vi "Icai 105 - Simultry11_Current Working Version.vi"() -> ()   [LabVIEW 2010]
uses:
  <vilib>/DAQmx/write.llb/DAQmx Write (Analog 1D Wfm NChan NSamp).vi
  <vilib>/DAQmx/write.llb/DAQmx Write (Digital 1D Bool 1Chan 1Samp).vi
  <vilib>/DAQmx/write.llb/DAQmx Write (Analog Wfm 1Chan NSamp).vi
  <vilib>/Waveform/WDTOps.llb/WDT Append Waveforms DBL.vi
  <vilib>/measure/matone.llb/Extract Single Tone Information 1 Chan.vi
  <vilib>/DAQmx/create/channels.llb/DAQmx Create Channel (DO-Digital Output).vi
  <vilib>/DAQmx/create/channels.llb/DAQmx Create Channel (AO-Voltage-Basic).vi
  <vilib>/DAQmx/configure/timing.llb/DAQmx Timing (Sample Clock).vi
  <vilib>/daqmx/miscellaneous.llb/DAQmx Fill In Error Info.vi
  <vilib>/measure/NI_MABase.lvlib
  <vilib>/measure/NI_MAPro.lvlib
  Program Files/National Instruments/LabVIEW 2010/resource/objmgr/daqmx.rc
panel:
  out "error out 2":errorcluster
  out "number of samples written per channel":u32
  out "detected frequency 2":dbl format="%.6p"
  out "SampClk.Timebase.Rate":dbl format="%^#_10g"
  in  "Freq Scale Factor":dbl=1.0 format="%#_12g"
  out "signal out":waveform(dbl)(graph)
  in  "lines":tag="Dev1/port0/line3"
  in  "Rising Logic Output Chan":tag="Dev1/ao2"
  in  "Mod Duration ms":i32=300
  in  "Samples (1Ms/s)":i32=500000
  out "min value":dbl
  in  "Falling Logic Output Chan":tag="Dev1/ao1"
  in  "FM Waveform Channel":tag="Dev1/ao3"
  out "error out":errorcluster caption="error out (DAQ)"
  out "Mod":dbl=118572.0
  out "Numeric 2":dbl=3900000.0 format="%#_7g"
  out "Numeric":dbl=3900000.0 format="%#_7g"
  in  "Pre-Trig Samples":ext=100.0 format="%.2f"
  out "?":dbl=579698.7113293351 format="%#_6f"
  out "#s":dbl=39524.02451426849
  in  "Time int":i32=30000
  in  "Sensitivity":u16(ring)=19 items=["2 nV/fA", "5 nV/fA", "10 nV/fA", "20 nV/fA", "50 nV/fA", "100 nV/fA", "200 nV/fA", "500 nV/fA", "1 uV/pA", "2 uV/pA", "5 uV/pA", "10 uV/pA", "20 uV/pA", "50 uV/pA", "100 uV/pA", "200 uV/pA", "500 uV/pA", "1 mV/nA", "2 mV/nA", "5 mV/nA", "10 mV/nA", "20 mV/nA", "50 mV/nA", "100 mV/nA", "200 mV/nA", "500 mV/nA", "1 V/uA"]
  in  "Detection Bandwidth":u16(ring)=6 items=["10 us/ 25 kHz", "30 us /8.33 kHz", "100 us/ 2.50 kHz", "300 us/ 833 Hz", "1 ms /250 Hz", "3 ms /83.3 Hz", "10 ms/ 25 Hz", "30 ms/ 8.33 Hz", "100 ms/ 2.50 Hz", "300 ms/ 0.833 Hz ", "1 s/ 0.250 Hz", "3 s/ 0.0833 Hz", "10 s/0.025 Hz"]
  in  "SR 830 GPIB Address":i32=8
  in  "Freq 2":dbl=2447.6 format="%_7g"
  out "Iterat #":dbl=10.0
  in  "Iteration":dbl=500.0
  in  "stop 2":bool
  in  "pulse":bool=TRUE
  in  "Start":ext=0.05
  out "?":waveform(dbl)[](graph)
  in  "amplitude 2":dbl=0.25 format="%0.2p"
  in  "?":T1(ring)
  in  "phase 2":dbl format="%.2p"
  in  "Offset 2":dbl=-0.0 format="%#_6p"
  in  "frequency 4":dbl=100.0 format="%0.2p"
  in  "?":T1(ring)=enum."Triangle Wave"
  in  "offset 4":dbl=-1.0 format="%0.2p"
  in  "phase 4":dbl=90.0 format="%.2p"
  in  "amplitude 4":dbl=1.0 format="%0.2p"
  in  "frequency 1":dbl=100.0 format="%0.2p"
  in  "amplitude 1":dbl=1.0 format="%0.2p"
  in  "sampling info 1":cluster{"Fs":dbl, "#s":dbl}={"Fs"=1000000.0, "#s"=2500.0} {"Fs" format="%.2p"}
  in  "?":T1(ring)=enum."Triangle Wave"
  in  "phase 1":dbl=-90.0 format="%.2p"
  in  "Offset 1":dbl format="%#_6p"
  in  "iterat":dbl
  out "CW":dbl=123571.0
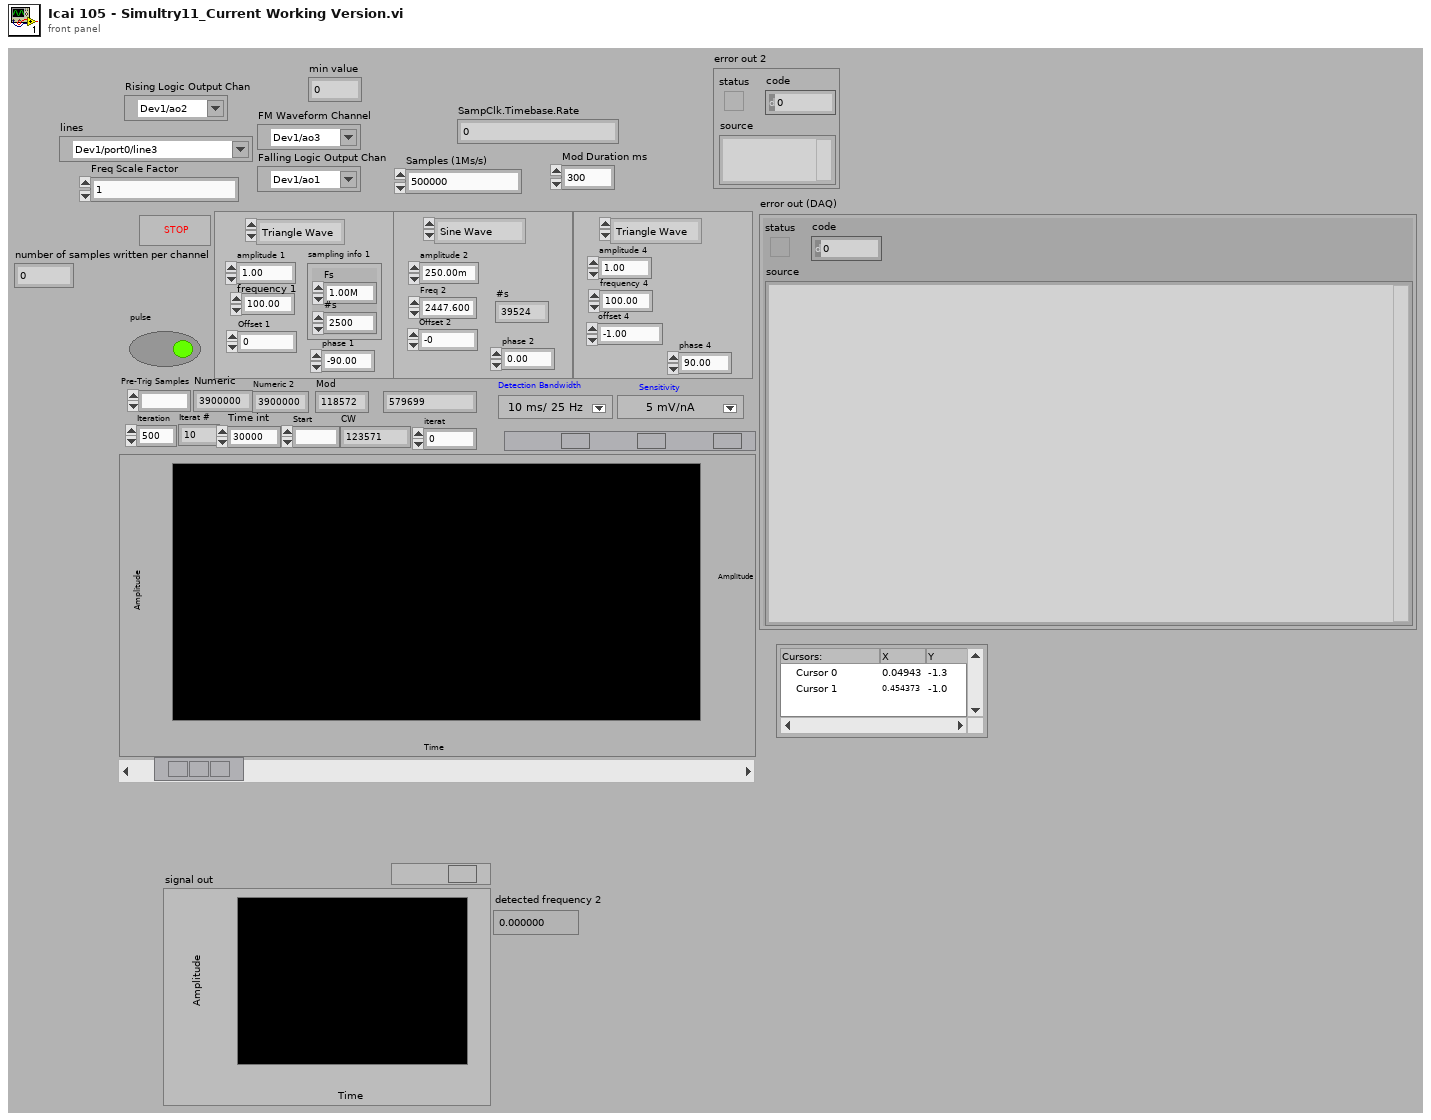
[diagram p1: front panel]
types:
  T1 = enum16{"Sine Wave", "Triangle Wave", "Square Wave", "Sawtooth Wave"}
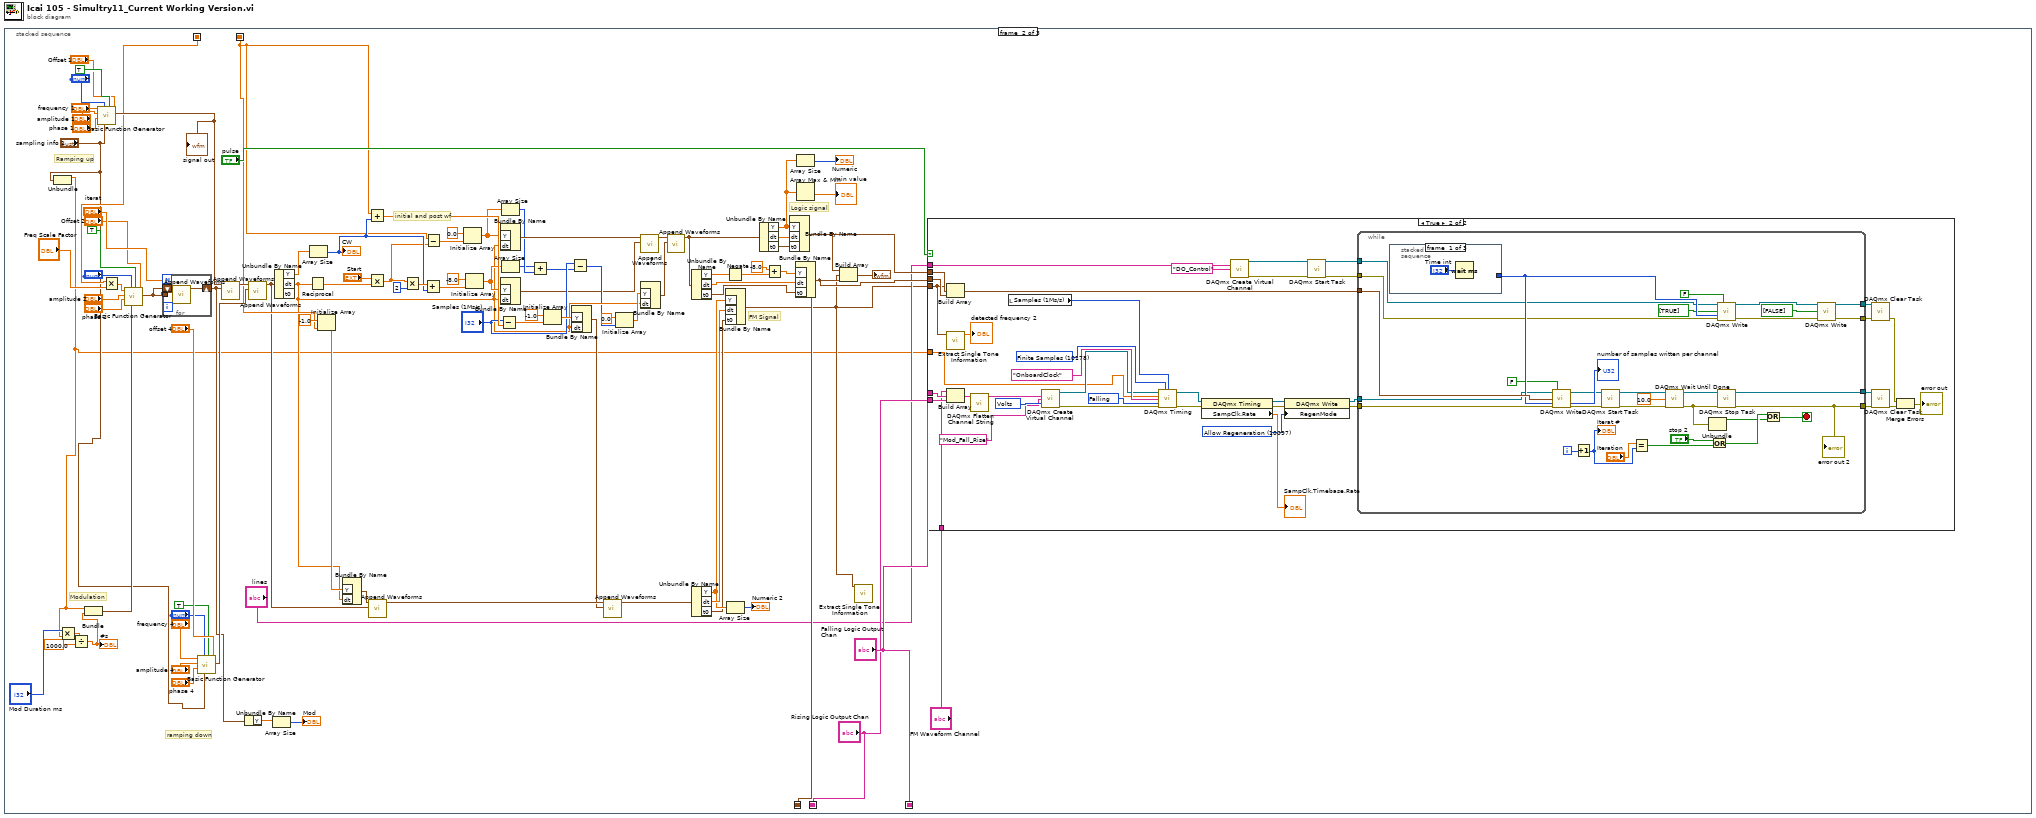
[diagram p0: block diagram]
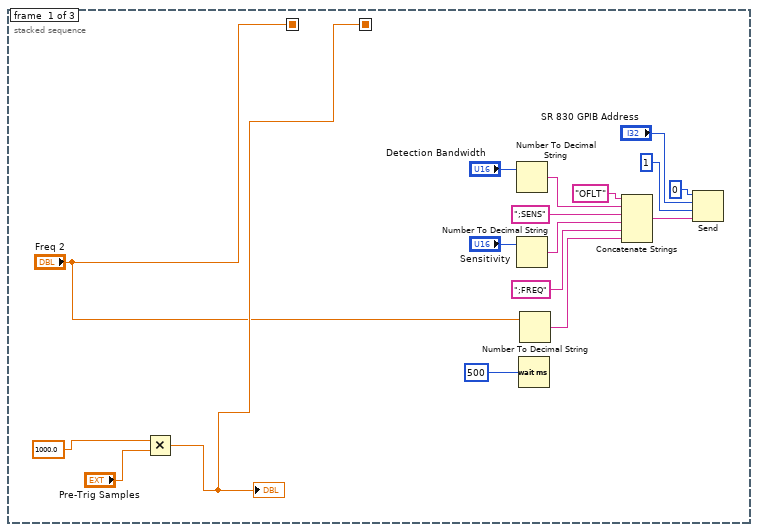
[diagram p2: hidden frame]
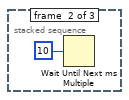
[diagram p4: hidden frame]
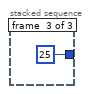
[diagram p5: hidden frame]
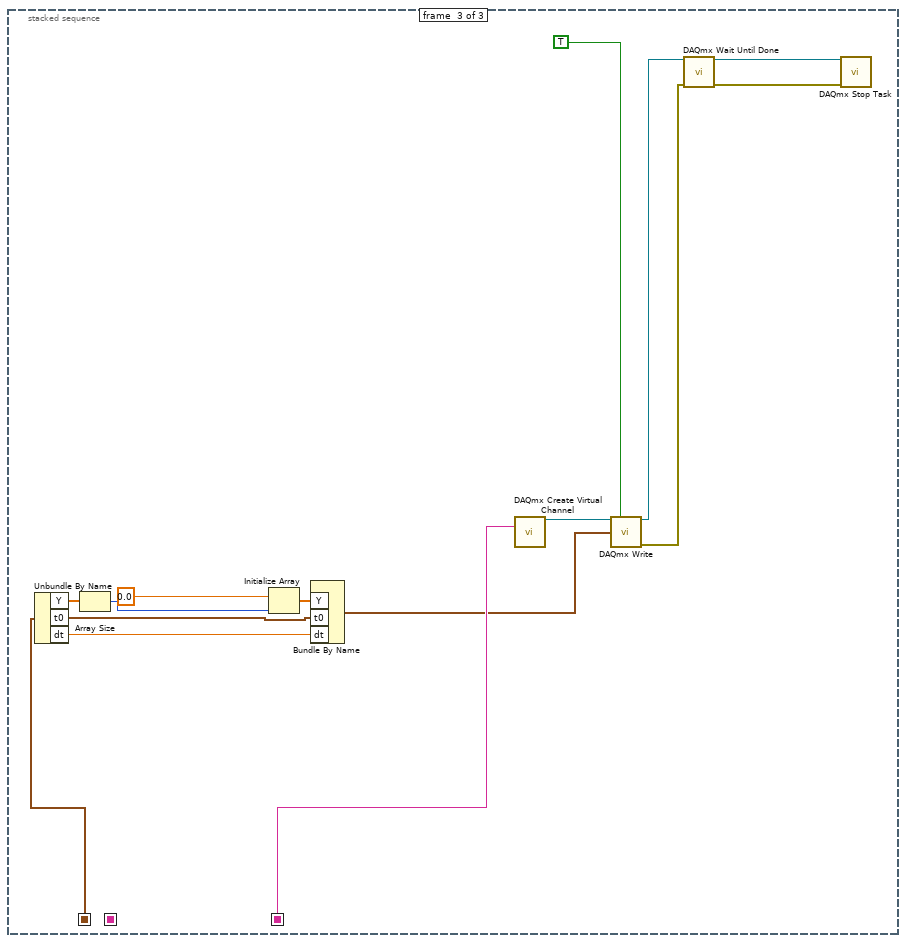
[diagram p6: hidden frame]
diagram:
  n1 = stacked-sequence {
    seq-local: ["Freq 2" _ _] -> [_ w23 _]
    seq-local: [w2 _ _] -> [_ w57 _]
    seq-local: [_ "Falling Logic Output Chan" _] -> [_ _ w194]
    seq-local: [_ "Rising Logic Output Chan" _] -> [_ _ _]
    seq-local: [_ w37 _] -> [_ _ w202]
    frame #0 {
      n2 = Multiply(x=1000.0 ("Fs 2"), y="Pre-Trig Samples") -> (x*y=w2:ext)
      "?" <- w2
      n3 = Number To Decimal String(number="Detection Bandwidth") -> (decimal integer string=w16:string)  [unwired: 1 out]
      n4 = Number To Decimal String(number="Sensitivity") -> (decimal integer string=w14:string)  [unwired: 1 out]
      n5 = Wait (ms)(milliseconds to wait=500) -> ()  [unwired: 1 out]
      n6 = Number To Decimal String(number="Freq 2") -> (decimal integer string=w5:string)  [unwired: 1 out]
      n7 = Concatenate Strings("OFLT", w16, ";SENS", w14, ";FREQ" ("string"), w5) -> (w13:string)
      n8 = Send(0:0 ("bus"), 2:"SR 830 GPIB Address", 3:i16 1 ("mode"), 5:w13) -> ()  [unwired: 1 in, 3 out]
    }
    frame #1 {
      # "initial and post wf"
      # "FM Signal"
      # "Logic signal"
      # "Ramping up"
      # "ramping down"
      # "Modulation"
      n9 = Unbundle("sampling info 1") -> ("Fs"=w18:dbl)  [unwired: 1 out]
      n10 = Multiply(x="Mod Duration ms", y=w18) -> (x*y=w29:dbl)
      n11 = Divide(x=w29, y=1000.0) -> (x/y=w27:dbl)
      "#s" <- w27
      n12 = Bundle("Fs"=w18, w27) -> (w61:cluster{"Fs":dbl, dbl})  [unwired: 1 out]
      n13 = call <vilib>:"Basic Function Generator.vi"("offset"="Offset 1", "reset signal"=TRUE, "sampling info"="sampling info 1", "signal type"="?", "phase"="phase 1", "amplitude"="amplitude 1", "frequency"="frequency 1") -> ("signal out"=w95:waveform(dbl))  [unwired: 2 in, 2 out]
      "signal out" <- w95
      n14 = Multiply(x=w23, y="Freq Scale Factor") -> (x*y=w22:dbl)
      n15 = call <vilib>:"Basic Function Generator.vi"("offset"="Offset 2", "reset signal"=TRUE, "sampling info"=w61, "signal type"="?", "phase"="phase 2", "amplitude"="amplitude 2", "frequency"=w22) -> ("signal out"=w25:waveform(dbl))  [unwired: 2 in, 2 out]
      n16 = for {
        N: "iterat" -> [_]
        shift-right: [w192] -> w50
        shift-left: w25 -> [w190]
        tunnel: w25 -> [w191]
        n17 = call-poly <vilib>:"Append Waveforms.vi"("waveform B"=w191, "waveform A"=w190) -> ("waveform out"=w192:waveform(dbl))  [unwired: 1 in, 8 out]
      }
      n18 = call <vilib>:"Basic Function Generator.vi"("offset"="offset 4", "reset signal"=TRUE, "sampling info"="sampling info 1", "signal type"="?", "phase"="phase 4", "amplitude"="amplitude 4", "frequency"="frequency 4") -> ("signal out"=w100:waveform(dbl))  [unwired: 2 in, 2 out]
      n19 = call-poly <vilib>:"Append Waveforms.vi"("waveform B"=w50, "waveform A"=w95) -> ("waveform out"=w94:waveform(dbl))  [unwired: 1 in, 8 out]
      n20 = Unbundle By Name(w50) -> ("Y"=w51:dbl[])
      n21 = call-poly <vilib>:"Append Waveforms.vi"("waveform B"=w100, "waveform A"=w94) -> ("waveform out"=w33:waveform(dbl))  [unwired: 1 in, 8 out]
      n22 = Array Size(array=w51) -> (size(s)=→"Mod":i32)
      n23 = Unbundle By Name(w33) -> ("Y"=w96:dbl[], "dt"=w56:dbl)  [unwired: 1 out]
      n24 = Reciprocal(x=w56) -> (1/x=w58:dbl)
      n25 = Array Size(array=w96) -> (size(s)=w78:i32)
      "CW" <- w78
      n26 = Initialize Array(-1.0 ("DC level"), w57) -> (w85:dbl[])
      n27 = Bundle By Name("Y"=w85, "dt"=w56) -> (w98:waveform(dbl))  [unwired: 1 out]
      n28 = Add(x=w57, y=w78) -> (x+y=w83:ext)
      n29 = Multiply(x="Start", y=w58) -> (x*y=w71:ext)
      n30 = call-poly <vilib>:"Append Waveforms.vi"("waveform B"=w33, "waveform A"=w98) -> ("waveform out"=w99:waveform(dbl))  [unwired: 1 in, 8 out]
      n31 = Multiply(x=w71, y=2) -> (x*y=w79:ext)
      n32 = Add(x=w79, y=w78) -> (x+y=w60:ext)
      n33 = Subtract(x=w57, y=w71) -> (x-y=w72:ext)
      n34 = Initialize Array(0.0 ("Trigger down"), w72) -> (w70:dbl[])
      n35 = Initialize Array(-8.0 ("Trigger up"), w60) -> (w69:dbl[])
      n36 = Subtract(x="Samples (1Ms/s)", y=w83) -> (x-y=w82:ext)
      n37 = Bundle By Name("Y"=w70, "dt"=w56) -> (w74:waveform(dbl))  [unwired: 1 out]
      n38 = Bundle By Name("Y"=w69, "dt"=w56) -> (w31:waveform(dbl))  [unwired: 1 out]
      n39 = Array Size(array=w70) -> (size(s)=w68:i32)
      n40 = Array Size(array=w69) -> (size(s)=w67:i32)
      n41 = Add(x=w67, y=w68) -> (x+y=w66:i32)
      n42 = Initialize Array(-1.0 ("DC level"), w82) -> (w81:dbl[])
      n43 = Subtract(x="Samples (1Ms/s)", y=w66) -> (x-y=w32:i32)
      n44 = Bundle By Name("Y"=w81, "dt"=w56) -> (w80:waveform(dbl))  [unwired: 1 out]
      n45 = call-poly <vilib>:"Append Waveforms.vi"("waveform B"=w80, "waveform A"=w99) -> ("waveform out"=w88:waveform(dbl))  [unwired: 1 in, 8 out]
      n46 = Initialize Array(0.0 ("Trigger down"), w32) -> (w75:dbl[])
      n47 = Bundle By Name("Y"=w75, "dt"=w56) -> (w73:waveform(dbl))  [unwired: 1 out]
      n48 = call-poly <vilib>:"Append Waveforms.vi"("waveform B"=w31, "waveform A"=w74) -> ("waveform out"=w91:waveform(dbl))  [unwired: 1 in, 8 out]
      n49 = call-poly <vilib>:"Append Waveforms.vi"("waveform B"=w73, "waveform A"=w91) -> ("waveform out"=w48:waveform(dbl))  [unwired: 1 in, 8 out]
      n50 = Unbundle By Name(w48) -> ("Y"=w47:dbl[], "dt"=w42:dbl, "t0"=w43:timestamp)
      n51 = Unbundle By Name(w88) -> ("Y"=w53:dbl[], "dt"=w87:dbl, "t0"=w30:timestamp)
      n52 = Bundle By Name("Y"=w53, "dt"=w87, "t0"=w30) -> (w24:waveform(dbl))  [unwired: 1 out]
      n53 = Negate(x=w47) -> (-x=w45:dbl[])
      n54 = Array Size(array=w53) -> (size(s)=→"Numeric 2":i32)
      n55 = Unbundle By Name(w48) -> ("Y"=w49:dbl[], "dt"=w89:dbl, "t0"=w44:timestamp)
      n56 = Add(x=-8.0, y=w45) -> (x+y=w41:dbl[])
      n57 = Bundle By Name("Y"=w49, "dt"=w89, "t0"=w44) -> (w36:waveform(dbl))  [unwired: 1 out]
      n58 = Bundle By Name("Y"=w41, "dt"=w42, "t0"=w43) -> (w37:waveform(dbl))  [unwired: 1 out]
      n59 = Array Size(array=w49) -> (size(s)=→"Numeric":i32)
      n60 = Array Max & Min(array=w49) -> (min value=→"min value":dbl)  [unwired: 3 out]
      n61 = Build Array(w36, w24, w37) -> (→"?":waveform(dbl)[])
      n62 = call-poly <vilib>:"Extract Single Tone Information.vi"("time signal in"=w24) -> ()  [unwired: 5 in, 6 out]
      n63 = case shown="True" "pulse" {
        tunnel: w24 -> [_ w133]
        tunnel: w36 -> [_ w151]
        tunnel: w37 -> [_ w135]
        tunnel: "Falling Logic Output Chan" -> [_ w131]
        tunnel: "Rising Logic Output Chan" -> [_ w130]
        tunnel: "lines" -> [_ w149]
        tunnel: "FM Waveform Channel" -> [_ w126]
        tunnel: w18 -> [_ w117]
        frame False {
        }
        frame True {
          w121 = 10097 items=["Allow Regeneration"=10097, "Do Not Allow Regeneration"=10158] ("RegenMode")
          w139 = 10348 items=["Volts"=10348, "From Custom Scale"=10065] ("units")
          w152 = 10178 items=["Finite Samples"=10178, "Continuous Samples"=10123, "Hardware Timed Single Point"=12522] ("sample mode")
          w153 = 10171 items=["Rising"=10280, "Falling"=10171] ("active edge")
          n64 = Build Array(w133, w151, w135) -> (w150:waveform(dbl)[])
          n65 = call-poly <vilib>:"Extract Single Tone Information.vi"("time signal in"=w133) -> ("detected frequency"=→"detected frequency 2":dbl)  [unwired: 5 in, 5 out]
          n66 = Build Array(w126, w131, w130) -> (w132:tag[])
          n67 = call <vilib>:"DAQmx Flatten Channel String.vi"("names in"=w132) -> ("names out"=w127:string)  [unwired: 13 in, 1 out]
          n68 = local read "Samples (1Ms/s)"() -> (w146:i32)
          n69 = call-poly <vilib>:"DAQmx Create Virtual Channel.vi"("physical channels"=w127, "name to assign"="Mod_Fall_Rise", "units"=w139) -> ("task out"=w129:refnum<k21>, "error out"=w128:errorcluster)  [unwired: 11 in]
          n70 = call-poly <vilib>:"DAQmx Timing.vi"("task/channels in"=w129, "sample mode"=w152, "samples per channel"=w146, "rate"=w117, "source"=tag "OnboardClock", "active edge"=w153, "error in"=w128) -> ("task out"=w138:refnum<k21>, "error out"=w137:errorcluster)  [unwired: 7 in]
          n71 = property class="DAQmx Timing"(reference=w138, error in=w137) -> (reference out=w125:refnum<k21>, error out=w124:errorcluster, "SampClk.Rate"=→"SampClk.Timebase.Rate":dbl)
          n72 = call-poly <vilib>:"DAQmx Create Virtual Channel.vi"("lines"=w149, "name to assign"="DO_Control") -> ("task out"=w145:refnum<k21>, "error out"=w140:errorcluster)  [unwired: 12 in]
          n73 = property class="DAQmx Write"(reference=w125, error in=w124, "RegenMode"=w121) -> (reference out=w122:refnum<k21>, error out=w123:errorcluster)
          n74 = call <vilib>:"DAQmx Start Task.vi"("task/channels in"=w145, "error in"=w140) -> ("task out"=w148:refnum<k21>, "error out"=w147:errorcluster)  [unwired: 12 in]
          n75 = while {
            tunnel: w150 -> [w181]
            tunnel: w148 -> [w179]
            tunnel: w147 -> [w177]
            tunnel: [w172] -> w143
            tunnel: [w171] -> w144
            tunnel: w122 -> [w170]
            tunnel: w123 -> [w169]
            tunnel: [w155] -> w119
            tunnel: [w156] -> w120
            i -> [w184]
            stop <- w163 stop-if-true
            n76 = stacked-sequence {
              tunnel: [_ _ 25 ("timeout (s)")] -> w180
              frame #0 {
                n77 = Wait (ms)(milliseconds to wait="Time int") -> ()  [unwired: 1 out]
              }
              frame #1 {
                n78 = Wait Until Next ms Multiple(millisecond multiple=u32 10) -> ()  [unwired: 1 out]
              }
              frame #2 {
              }
            }
            n79 = call-poly <vilib>:"DAQmx Write.vi"("task/channels in"=w170, "auto start"=FALSE, "data"=w181, "timeout"=w180, "error in"=w169) -> ("task out"=w160:refnum<k21>, "number of samples written per channel"=→"number of samples written per channel":u32, "error out"=w159:errorcluster)  [unwired: 8 in]
            n80 = Increment(x=w184) -> (x+1=w182:i32)
            "Iterat #" <- w182
            n81 = call <vilib>:"DAQmx Start Task.vi"("task/channels in"=w160, "error in"=w159) -> ("task out"=w157:refnum<k21>, "error out"=w158:errorcluster)  [unwired: 12 in]
            n82 = Equal?(x="Iteration", y=w182) -> (x = y?=w186:bool)
            n83 = call <vilib>:"DAQmx Wait Until Done.vi"("task/channels in"=w157, "timeout (sec)"=10.0, "error in"=w158) -> ("task out"=w162:refnum<k21>, "error out"=w161:errorcluster)  [unwired: 11 in]
            n84 = Unbundle(w161) -> ("status"=w164:bool)  [unwired: 2 out]
            n85 = Or(x="stop 2", y=w186) -> (x .or. y?=w165:bool)
            n86 = call-poly <vilib>:"DAQmx Write.vi"("task/channels in"=w179, "auto start"=FALSE, "data"=bool[] [TRUE], "timeout"=w180, "error in"=w177) -> ("task out"=w175:refnum<k21>, "error out"=w173:errorcluster)  [unwired: 8 in, 1 out]
            n87 = call <vilib>:"DAQmx Stop Task.vi"("task/channels in"=w162, "error in"=w161) -> ("task out"=w156:refnum<k21>, "error out"=w155:errorcluster)  [unwired: 12 in]
            "error out 2" <- w155
            n88 = Or(x=w165, y=w164) -> (x .or. y?=w163:bool)
            n89 = call-poly <vilib>:"DAQmx Write.vi"("task/channels in"=w175, "data"=bool[] [FALSE], "error in"=w173) -> ("task out"=w171:refnum<k21>, "error out"=w172:errorcluster)  [unwired: 10 in, 1 out]
          }
          n90 = call <vilib>:"DAQmx Clear Task.vi"("task in"=w144, "error in"=w143) -> ("error out"=w142:errorcluster)  [unwired: 13 in]
          n91 = call <vilib>:"DAQmx Clear Task.vi"("task in"=w120, "error in"=w119) -> ("error out"=w118:errorcluster)  [unwired: 13 in]
          n92 = Merge Errors(w142, w118) -> (→"error out":errorcluster)
        }
      }
    }
    frame #2 {
      n93 = Unbundle By Name(w202) -> ("Y"=w199:dbl[], "t0"=w201:timestamp, "dt"=w200:dbl)
      n94 = Array Size(array=w199) -> (size(s)=w198:i32)
      n95 = Initialize Array(0.0 ("element"), w198) -> (w196:dbl[])
      n96 = Bundle By Name("Y"=w196, "t0"=w201, "dt"=w200) -> (w193:waveform(dbl))  [unwired: 1 in]
      n97 = call-poly <vilib>:"DAQmx Create Virtual Channel.vi"("physical channels"=w194) -> ("task out"=w195:refnum<k21>)  [unwired: 13 in, 1 out]
      n98 = call-poly <vilib>:"DAQmx Write.vi"("task/channels in"=w195, "auto start"=TRUE, "data"=w193) -> ("task out"=w203:refnum<k21>, "error out"=w206:errorcluster)  [unwired: 10 in, 1 out]
      n99 = call <vilib>:"DAQmx Wait Until Done.vi"("task/channels in"=w203, "error in"=w206) -> ("task out"=w205:refnum<k21>, "error out"=w207:errorcluster)  [unwired: 12 in]
      n100 = call <vilib>:"DAQmx Stop Task.vi"("task/channels in"=w205, "error in"=w207) -> ()  [unwired: 12 in, 2 out]
    }
  }
